vi "CAN Jaguar Config Max Output Voltage.vi"(8 "error in (no error)":errorcluster, 10 "Maximum Output Voltage":dbl, 11 "CAN Jaguar Ref":T1={"Device Number"=0, "Control Mode"=enum."Percent VBus", "Inverted"=FALSE, "Semaphore"=refnum, "Max Vout"=12.0, "DevStatus"={"status"=FALSE, "code"=0, "source"=""}}) -> (0 "error out":errorcluster, 3 "CAN Jaguar Ref Out":T1={"Device Number"=0, "Control Mode"=enum."Percent VBus", "Inverted"=FALSE, "Semaphore"=refnum, "Max Vout"=12.0, "DevStatus"={"status"=FALSE, "code"=0, "source"=""}})   [LabVIEW 2009, in "CAN.lvlib"]
uses:
  CAN.lvlib
  SubVIs/CAN Motor Message IDs.ctl
  SubVIs/CAN Jaguar Control Mode.ctl
  SubVIs/CAN Jaguar Ref.ctl
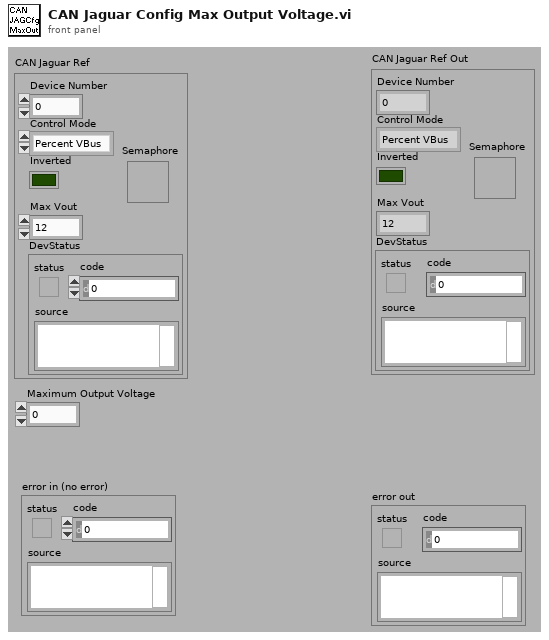
[diagram p1: front panel]
types:
  T1 = typedef "CAN.lvlib/CAN Jaguar Ref.ctl" = cluster{"Device Number":u8, "Control Mode":T2, "Inverted":bool, "Semaphore":T3, "Max Vout":dbl, "DevStatus":errorcluster}
  T2 = typedef "CAN.lvlib/CAN Jaguar Control Mode.ctl" = enum16{"Percent VBus", "Speed", "Position", "Current"}
  T3 = typedef "Semaphore RefNum" = refnum<k1>
  T4 = enum16{"big-endian, network order", "native, host order", "little-endian"}
  T5 = typedef "CAN.lvlib/CAN Motor Message IDs.ctl" = u32
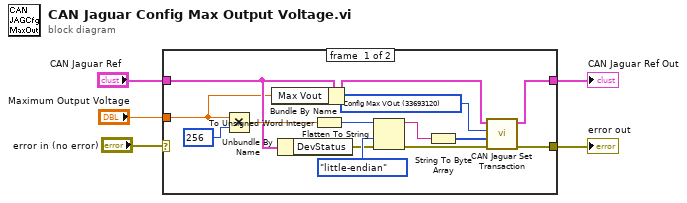
[diagram p0: block diagram]
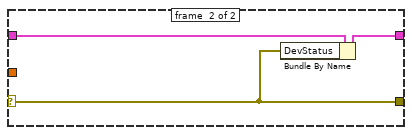
[diagram p2: hidden frame]
diagram:
  n1 = case shown="No Error" "error in (no error)" {
    selector: "error in (no error)" -> [_ w20]
    tunnel: [w12 w20] -> w5
    tunnel: [w10 w21] -> w3
    tunnel: "CAN Jaguar Ref" -> [w11 w22]
    tunnel: "Maximum Output Voltage" -> [w6 _]
    frame #0 {
      w9 = T5 33693120 items=["Volt Enable"=33685504, "Volt Disable"=33685568, "Volt Set"=33685632, "Volt Set Ramp"=33685696, "Speed Enable"=33686528, "Speed Disable"=33686592, "Speed Set"=33686656, "Speed P"=33686720, "Speed I"=33686784, "Speed D"=33686848, "Speed Ref"=33686912, "Position Enable"=33688576, "Position Disable"=33688640, "Position Set"=33688704, "Position P"=33688768, "Position I"=33688832, "Position D"=33688896, "Position Ref"=33688960, "Current Enable"=33689600, "Current Disable"=33689664, "Current Set"=33689728, "Current P"=33689792, "Current I"=33689856, "Current D"=33689920, "Status VOut"=33690624, "Status VBus"=33690688, "Status Current"=33690752, "Status Temp"=33690816, "Status Position"=33690880, "Status Speed"=33690944, "Status Limit"=33691008, "Status Fault"=33691072, "Status Power"=33691136, "Config Num Brushes"=33692672, "Config Encoder Lines"=33692736, "Config Pot Turns"=33692800, "Config Brake Coast"=33692864, "Config Limit Mode"=33692928, "Config Limit Fwd"=33692992, "Config Limit Rev"=33693056, "Config Max VOut"=33693120, "Config Fault Time"=33693184, "Motor Ack"=33693696] ("CAN Motor Message IDs")
      n2 = Multiply(x=w6, y=256) -> (x*y=w16:dbl)
      n3 = Bundle By Name(cluster=w11, "Max Vout"=w6) -> (w7:T1)
      n4 = Unbundle By Name(w11) -> ("DevStatus"=w14:errorcluster)
      n5 = To Unsigned Word Integer(number=w16) -> (unsigned 16bit integer=w17:u16)
      n6 = Flatten To String(anything=w17, byte order (0:big-endian, network order)=T4."little-endian", error in (no error)=w14) -> (data string=w18:string, error out=w13:errorcluster)  [unwired: 2 out]
      n7 = String To Byte Array(string=w18) -> (unsigned byte array=w8:u8[])
      n8 = call "CAN Jaguar Set Transaction.vi"("error in"=w13, "Data"=w8, "Message ID"=w9, "CAN Jaguar Ref"=w7) -> ("error out"=w12:errorcluster, "CAN Jaguar Ref Out"=w10:T1)  [unwired: 6 out]
    }
    frame #1 {
      n9 = Bundle By Name(cluster=w22, "DevStatus"=w20) -> (w21:T1)
    }
  }
  "CAN Jaguar Ref Out" <- w3
  "error out" <- w5
